vi "write module object.vi"(8 "error in":errorcluster, 10 "module information":T1 {"product ID" format="%.0x"}, 11 "Module in":refnum<class "Module.lvclass">) -> (0 "error out":errorcluster, 3 "Module out":refnum<class "Module.lvclass">)   [LabVIEW 2014, in "SMI.lvlib" / "Module.lvclass"]
uses:
  Module.lvclass
  module information.ctl
  Device/write serial number.vi
  Device/write product ID.vi
  Device/write product name.vi
  Device/write vendor name.vi
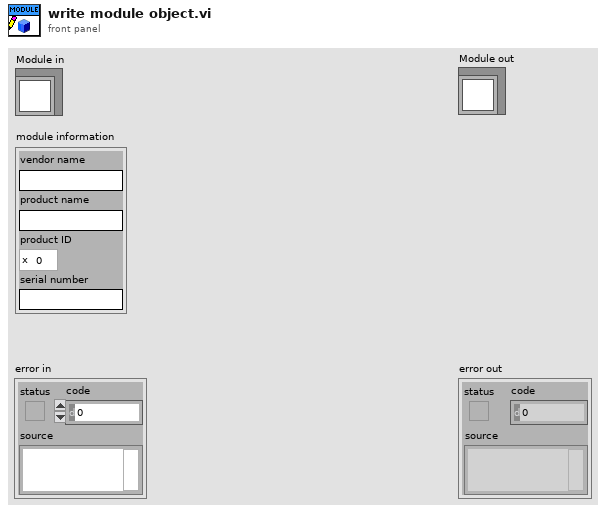
[diagram p1: front panel]
types:
  T1 = typedef "SMI.lvlib/Module.lvclass/module information.ctl" = cluster{"vendor name":string, "product name":string, "product ID":u16, "serial number":string}
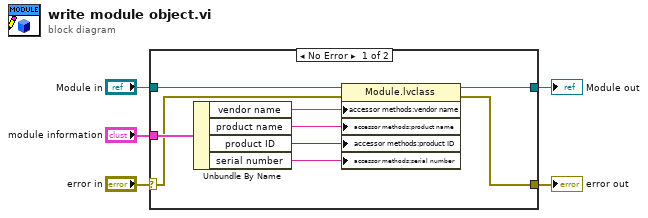
[diagram p0: block diagram]
diagram:
  n1 = case shown="No Error" "error in" {
    selector: "error in" -> [w7 w16]
    tunnel: [w6 w16] -> w4
    tunnel: [w13 w15] -> w1
    tunnel: "Module in" -> [w14 w15]
    tunnel: "module information" -> [w12 _]
    frame No Error {
      n2 = Unbundle By Name(w12) -> ("vendor name"=w11:string, "product name"=w10:string, "product ID"=w9:u16, "serial number"=w8:string)
      n3 = property class="Module.lvclass"(reference=w14, error in=w7, "accessor methods:vendor name"=w11, "accessor methods:product name"=w10, "accessor methods:product ID"=w9, "accessor methods:serial number"=w8) -> (reference out=w13:refnum<class "Module.lvclass">, error out=w6:errorcluster)
    }
    frame Error {
    }
  }
  "error out" <- w4
  "Module out" <- w1
